vi "DM get burst by name.vi"(8 "error in (no error)":errorcluster, 10 "Burst name":string, 11 "group":string) -> (0 "error out":errorcluster, 3 "TX burst":refnum<class "mmWave data.lvclass">)   [LabVIEW 2019, in "DataManagment.lvlib"]
uses:
  DataManagment.lvlib
  SubVIs/mmWave data_class/mmWave data.lvclass
  DM get burst parameters.ctl
  <vilib>/Utility/error.llb/Error Cluster From Error Code.vi
  <vilib>/ErrorRing/Error Ring.xnode
  <vilib>/addons/_JKI.lib/Serialization/JSON/JKI JSON Serialization.lvlib
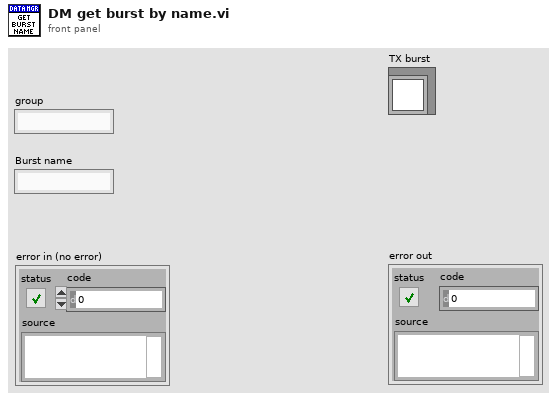
[diagram p1: front panel]
types:
  T1 = typedef "DataManagment.lvlib/DM get burst parameters.ctl" = cluster{"group":string, "bursts":string[]}
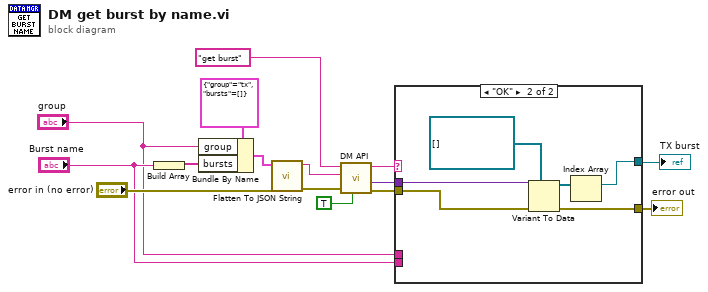
[diagram p0: block diagram]
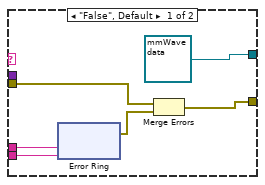
[diagram p2: hidden frame]
diagram:
  n1 = Build Array("Burst name") -> (w7:string[])
  n2 = Bundle By Name(cluster=T1 {"group"="tx", "bursts"=[]} ("Cluster"), "group"="group", "bursts"=w7) -> (w6:T1)
  n3 = call <vilib>:"Flatten To JSON String.vi"("error in (no error)"="error in (no error)", "Variant"=w6) -> ("error out"=w4:errorcluster, "JSON String"=w3:string)  [unwired: 8 in]
  n4 = call "DM API.vi"("response"=TRUE, "error in (no error)"=w4, "parameters"=w3, "message"="get burst") -> ("error out"=w10:errorcluster, "data"=w12:variant, "status"=w13:string)  [unwired: 4 in, 1 out]
  n5 = case shown="\"OK\"" w13 {
    tunnel: w12 -> [_ w35]
    tunnel: [refnum<class "mmWave data.lvclass"> refnum ("mmWave data") w30] -> w11
    tunnel: [w19 w31] -> w9
    tunnel: w10 -> [w18 w32]
    tunnel: "Burst name" -> [w17 _]
    tunnel: "group" -> [w16 _]
    frame "False", Default {
      n6 = xnode "Error Ring"("parameter 0"=w16, "parameter 1"=w17) -> ("error out"=w20:errorcluster)
      n7 = Merge Errors(w18, w20) -> (w19:errorcluster)
    }
    frame "OK" {
      n8 = Variant To Data(error in=w32, type=refnum<class "mmWave data.lvclass">[] [] ("Array"), Variant=w35) -> (data=w33:refnum<class "mmWave data.lvclass">[], error out=w31:errorcluster)
      n9 = Index Array(array=w33) -> (element=w30:refnum<class "mmWave data.lvclass">)  [unwired: 1 in]
    }
  }
  "TX burst" <- w11
  "error out" <- w9
